vi "Combine Tags.vi"(8 "error in (no error)":errorcluster, 10 "Appended uData":refnum<class "uData.lvclass">, 11 "Base uData":refnum<class "uData.lvclass">) -> (0 "error out":errorcluster, 3 "Combined uData":refnum<class "uData.lvclass">, 4 "Overwritten Tags":string[](array[string]))   [LabVIEW 2023, in "uLib.lvlib" / "uData.lvclass"]
doc: "Combine all the tags from two uData objects into one uData objects.\nIf the same tag exist in both objects, the tag value from the appended object overwrites the values which are in the base object tags."
uses:
  uData.lvclass
  uData.lvclass/uData.ctl
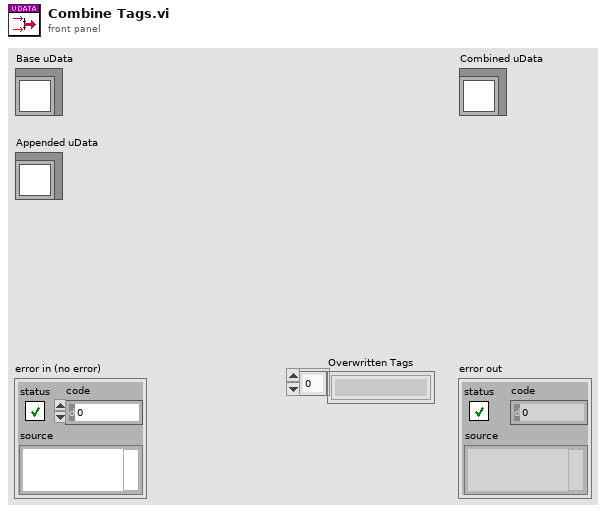
[diagram p1: front panel]
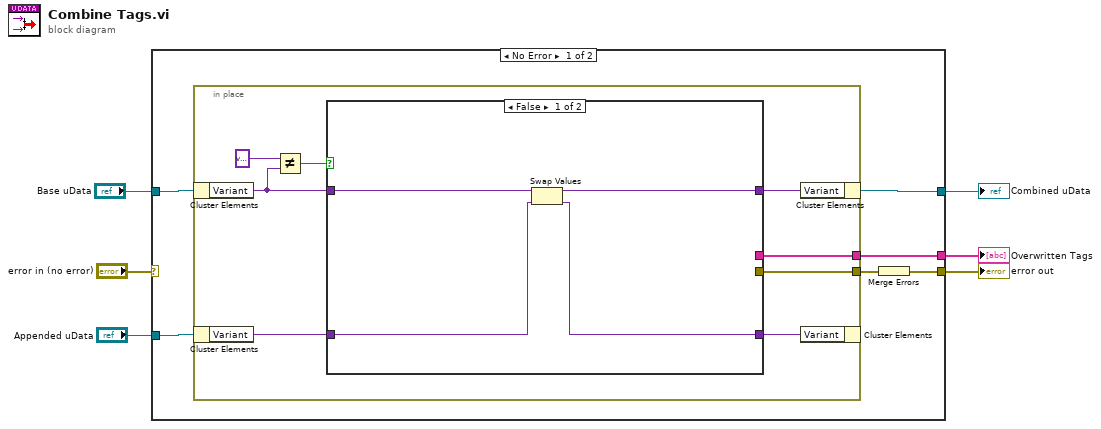
[diagram p0: block diagram]
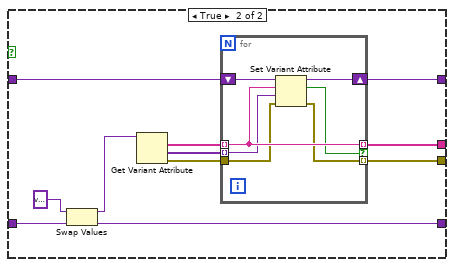
[diagram p2: hidden frame]
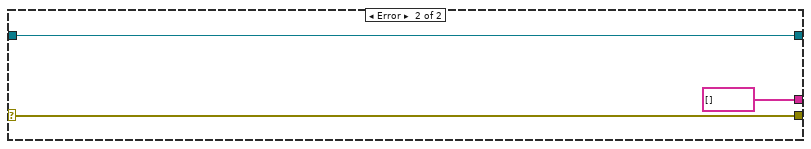
[diagram p3: hidden frame]
diagram:
  n1 = case shown="No Error" "error in (no error)" {
    selector: "error in (no error)" -> [_ w45]
    tunnel: "Base uData" -> [w12 w44]
    tunnel: "Appended uData" -> [w11 _]
    tunnel: [w7 w45] -> w3
    tunnel: [w10 w44] -> w2
    tunnel: [w9 string[] []] -> w1
    frame No Error {
      n2 = in-place {
        in-place-border: [w17] -> w9
        in-place-border: [w16] -> w8
        n3 = in-place-cluster #1(w12) -> ("Variant"=w14:variant)
        n4 = in-place-cluster #2(w11) -> ("Variant"=w19:variant)
        n5 = Not Equal?(x=variant, y=w14) -> (x != y?=w13:bool)
        n6 = case shown="False" w13 {
          tunnel: w14 -> [w23 w35]
          tunnel: [w24 w34] -> w20
          tunnel: w19 -> [w21 w32]
          tunnel: [w22 w31] -> w18
          tunnel: [_ w28] -> w17
          tunnel: [_ w25] -> w16
          frame False {
            n7 = Swap Values(12:w23, 14:w21) -> (1:w24:variant, 3:w22:variant)  [unwired: 1 in]
          }
          frame True {
            n8 = Swap Values(12:variant, 14:w32) -> (1:w29:variant, 3:w31:variant)  [unwired: 1 in]
            n9 = Get Variant Attribute(Variant=w29) -> (names=w33:string[], values=w27:variant[], error out=w26:errorcluster)  [unwired: 3 in, 1 out]
            n10 = for {
              shift-right: [w41] -> w34
              shift-left: w35 -> [w42]
              tunnel: w33 -> [w40] mode=indexing
              tunnel: [w40] -> w28 mode=indexing if=w38
              tunnel: w27 -> [w39] mode=indexing
              tunnel: w26 -> [w36]
              tunnel: [w37] -> w25 mode=indexing
              n11 = Set Variant Attribute(Variant=w42, name=w40, value=w39, error in=w36) -> (Variant out=w41:variant, replaced=w38:bool, error out=w37:errorcluster)
            }
          }
        }
        n12 = in-place-cluster #1("Variant"=w20) -> (w10:refnum<class "uData.lvclass">)
        n13 = in-place-cluster #2("Variant"=w18) -> ()  [unwired: 1 out]
      }
      n14 = Merge Errors(w8) -> (w7:errorcluster)
    }
    frame Error {
    }
  }
  "error out" <- w3
  "Combined uData" <- w2
  "Overwritten Tags" <- w1
